vi "Fakultaet und Produkt.vi"() -> ()   [LabVIEW 2017]
panel:
  out "Produkt":dbl
  out "n!":dbl
  in  "Faktor 2":dbl
  in  "Faktor 1":dbl
  in  "n":dbl
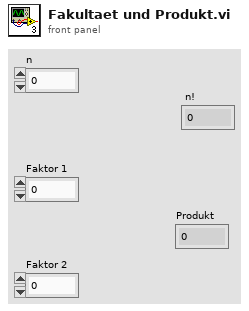
[diagram p1: front panel]
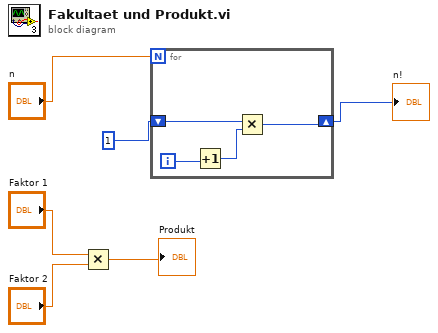
[diagram p0: block diagram]
diagram:
  n1 = Multiply(x="Faktor 1", y="Faktor 2") -> (x*y=→"Produkt":dbl)
  n2 = for {
    N: "n" -> [_]
    shift-right: [w7] -> w2
    shift-left: 1 -> [w8]
    i -> [w10]
    n3 = Increment(x=w10) -> (x+1=w9:i32)
    n4 = Multiply(x=w8, y=w9) -> (x*y=w7:i32)
  }
  "n!" <- w2
